vi "Modify Text Style.vi"(6 "Column # (0)":i32, 8 "error in":errorcluster, 9 "Status":string(combo), 10 "Tag(Current)":string, 11 "Tree Reference":refnum<vi>) -> (0 "error out":errorcluster, 3 "reference out":refnum<vi>)   [LabVIEW 2014, in "DSLV_Tree.lvlib"]
uses:
  DSLV_Tree.lvlib
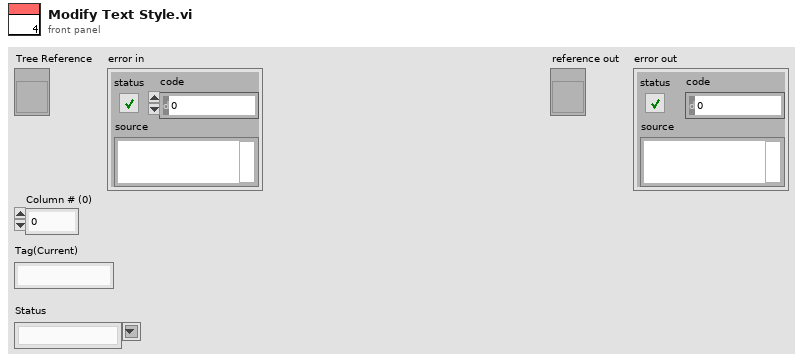
[diagram p1: front panel]
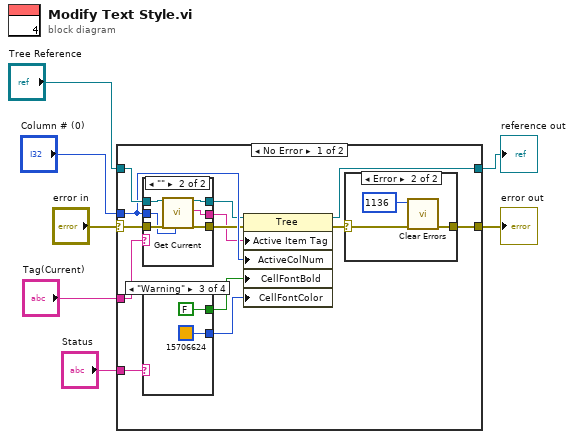
[diagram p0: block diagram]
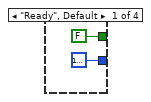
[diagram p3: hidden frame]
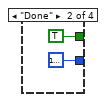
[diagram p4: hidden frame]
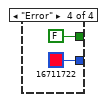
[diagram p5: hidden frame]
diagram:
  n1 = case shown="No Error" "error in" {
    selector: "error in" -> [w10 w42]
    tunnel: "Tag(Current)" -> [w20 _]
    tunnel: "Tree Reference" -> [w19 w43]
    tunnel: "Column # (0)" -> [w18 _]
    tunnel: "Status" -> [w14 _]
    tunnel: [w11 w43] -> w3
    tunnel: [w8 w42] -> w2
    frame No Error {
      n2 = case shown="\"\"" w20 {
        selector: w20 -> [w34 _]
        tunnel: [w35 w41] -> w17
        tunnel: w19 -> [w35 w40]
        tunnel: [w33 w39] -> w16
        tunnel: w10 -> [w33 w38]
        tunnel: [w34 w37] -> w15
        tunnel: w18 -> [_ w36]
        frame "False", Default {
        }
        frame "" {
          n3 = call "Get Current.vi"("Tree Reference In"=w40, "error in (no error)"=w38, "Column # (0)"=w36) -> ("Tree Reference Out"=w41:refnum<vi>, "Current Tag"=w37:string, "error out"=w39:errorcluster)  [unwired: 13 in, 1 out]
        }
      }
      n4 = case shown="\"Warning\"" w14 {
        tunnel: [FALSE TRUE FALSE FALSE] -> w13
        tunnel: [u32 16777222 ("Color Box") u32 16777222 ("Color Box") u32 15706624 ("Color Box") u32 16711722 ("Color Box")] -> w12
        frame "Ready", Default {
        }
        frame "Done" {
        }
        frame "Warning" {
        }
        frame "Error" {
        }
      }
      n5 = property on="Property Node" class="Tree"(reference=w17, error in=w16, "Active Item Tag"=w15, "ActiveColNum"=w18, "CellFontBold"=w13, "CellFontColor"=w12) -> (reference out=w11:refnum<vi>, error out=w9:errorcluster)
      n6 = case shown="Error" w9 {
        selector: w9 -> [w21 w23]
        tunnel: [w21 w22] -> w8
        frame No Error {
        }
        frame Error {
          n7 = call <vilib>:"Clear Errors.vi"("error in (no error)"=w23, "specific error code to clear (0: all)"=1136) -> ("error out"=w22:errorcluster)  [unwired: 4 in, 1 out]
        }
      }
    }
    frame Error {
    }
  }
  "reference out" <- w3
  "error out" <- w2
